vi "Vibrometer_Search.vi"(11 "VISA Refnum in":refnum<visa-resource-name>) -> (0 "error out":errorcluster, 2 "Success?":bool, 3 "VISA Refnum out":refnum<visa-resource-name>)   [LabVIEW 2022 SP3]
panel:
  out "find list":string[](array[string])
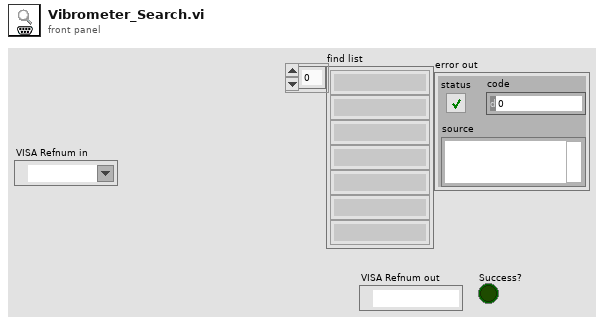
[diagram p1: front panel]
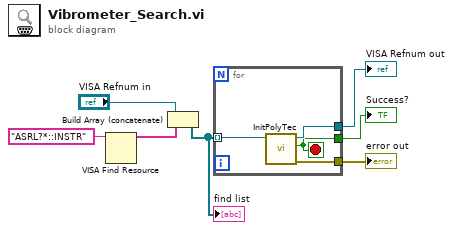
[diagram p0: block diagram]
diagram:
  n1 = VISA Find Resource(11:"ASRL?*::INSTR" ("expression (\"?*\")")) -> (3:w2:string[])  [unwired: 2 in, 2 out]
  n2 = Build Array (concatenate)("VISA Refnum in", w2) -> (w1:refnum<visa-resource-name>[])
  "find list" <- w1
  n3 = for {
    tunnel: w1 -> [w11] mode=indexing
    tunnel: [w10] -> w6
    tunnel: [w9] -> w4
    tunnel: [w8] -> w5
    stop <- w8 stop-if-true
    n4 = call "InitPolyTec.vi"("VISA Refnum in"=w11) -> ("error out"=w9:errorcluster, "Success?"=w8:bool, "VISA Refnum out"=w10:refnum<visa-resource-name>)  [unwired: 8 in]
  }
  "VISA Refnum out" <- w6
  "Success?" <- w5
  "error out" <- w4
